vi "ShooterSpeedRegulateV2 Debug.vi"(0 "Shooter Speed":T2(ring)) -> (4 "ALL GOOD":bool, 10 "Motor 1 Output":dbl)   [LabVIEW 2012]
uses:
  Robot Global Data.vi
  Max'sToolKit/ConvertVoltageToPercentVbs.vi
  <vilib>/addons/control/pid/pid.llb/PID (DBL).vi
  <vilib>/addons/control/pid/NI_PID_pid.lvlib
panel:
  in  "Use PID":bool
  out "Waveform Chart":cluster{dbl, "upper limit":dbl, dbl}(graph)
  in  "Feed Foward \nVoltage":dbl format="%_6g"
  in  "PID gains":T1
  out "Motor Voltage":dbl
  out "Error":dbl
  in  "Reset Shooter PID":bool
  out "Loop Rate (Hz)":dbl
  out "Array Index":dbl
  out "Wheel 1 RPS":dbl
  out "W1 Target RPS":dbl
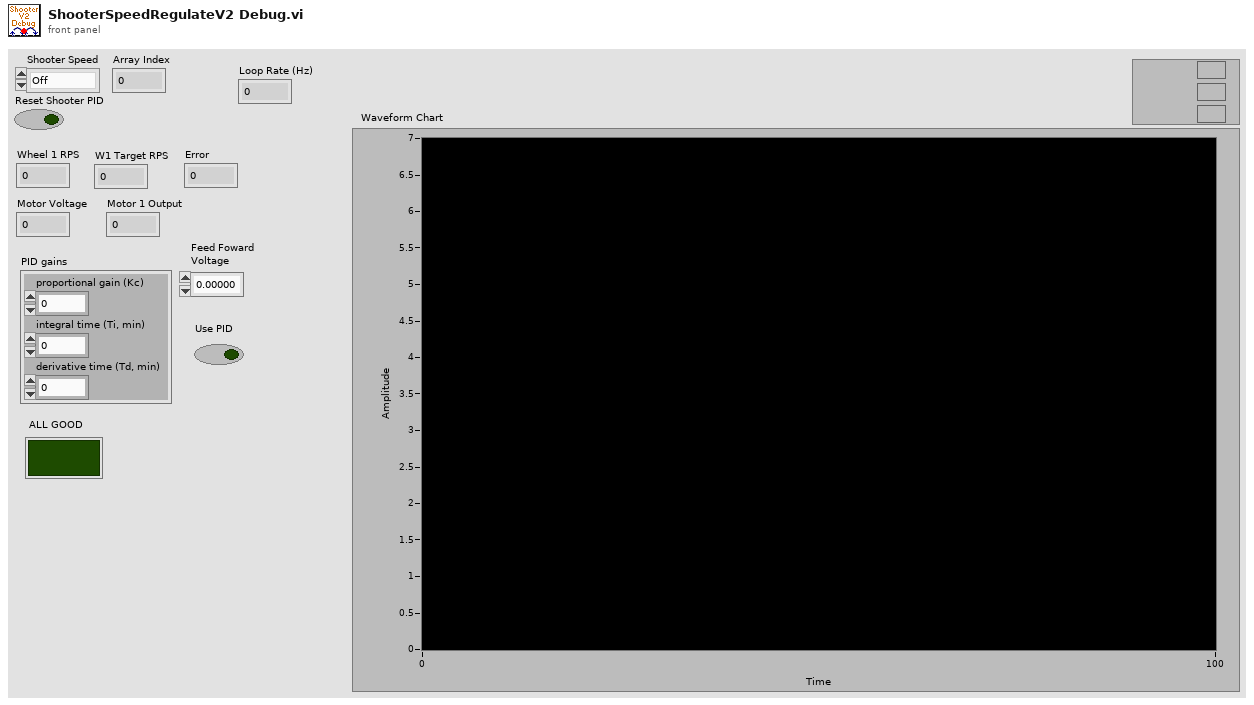
[diagram p1: front panel]
types:
  T1 = cluster{"proportional gain (Kc)":dbl, "integral time (Ti, min)":dbl, "derivative time (Td, min)":dbl}
  T2 = enum16{"Off", "2pt Key Shot", "3pt Key Shot", "Back Shot", "Fender Shot", "Key Close", "Key Far"}
  T3 = typedef "WPI_EncoderDevRef.ctl" = cluster{"DevStatus":errorcluster, "EncoderIndex":T4, "CounterIndex":T5, "DistancePerCount":dbl, "Decoding Type":T6}
  T4 = typedef "FPGA_EncoderIdx.ctl" = enum8{"Enc 0", "Enc 1", "Enc 2", "Enc 3", "Invalid"}
  T5 = typedef "FPGA_CounterCtrSystemIndex.ctl" = enum8{"Ctr 0", "Ctr 1", "Ctr 2", "Ctr 3", "Ctr 4", "Ctr 5", "Ctr 6", "Ctr 7", "Invalid"}
  T6 = typedef "WPI_EncoderType.ctl" = enum16{"1x", "2x", "4x"}
  T7 = typedef "WPI_MotorControlDeviceRef.ctl" = cluster{"DeviceStatus":errorcluster, "Type":enum16{"PWM", "CAN"}, "PWM":cluster{"Digital Module":T8, "PWM Channel":T9, "DeadBand":T10}, "CAN":cluster{"Device Number":u8, "Control Mode":T11, "Semaphore":T12, "Max Vout":dbl}, "Invert":bool, "TransformRef":T13, "InvTransformRef":T13}
  T8 = typedef "FPGA_TypedefDigitalModule.ctl" = enum16{"Digital Module 1", "Digital Module 2"}
  T9 = typedef "FPGA_DIOPWMChannel.ctl" = enum8{"PWM 1", "PWM 2", "PWM 3", "PWM 4", "PWM 5", "PWM 6", "PWM 7", "PWM 8", "PWM 9", "PWM 10", "Invalid"}
  T10 = typedef "WPI_PWMDeadband.ctl" = cluster{"Name":string, "maxPositivePwm":i32, "minPositivePwm":i32, "centerPwm":i32, "maxNegativePwm":i32, "minNegativePwm":i32, "angularRange":u16}
  T11 = typedef "WPI_CANJaguar_ControlMode.ctl" = enum8{"Percent VBus", "Current", "Speed", "Position", "Voltage"}
  T12 = typedef "Semaphore RefNum" = refnum<k1>
  T13 = typedef "WPI_PWMTransform_ConPane.ctl" = refnum<vi>
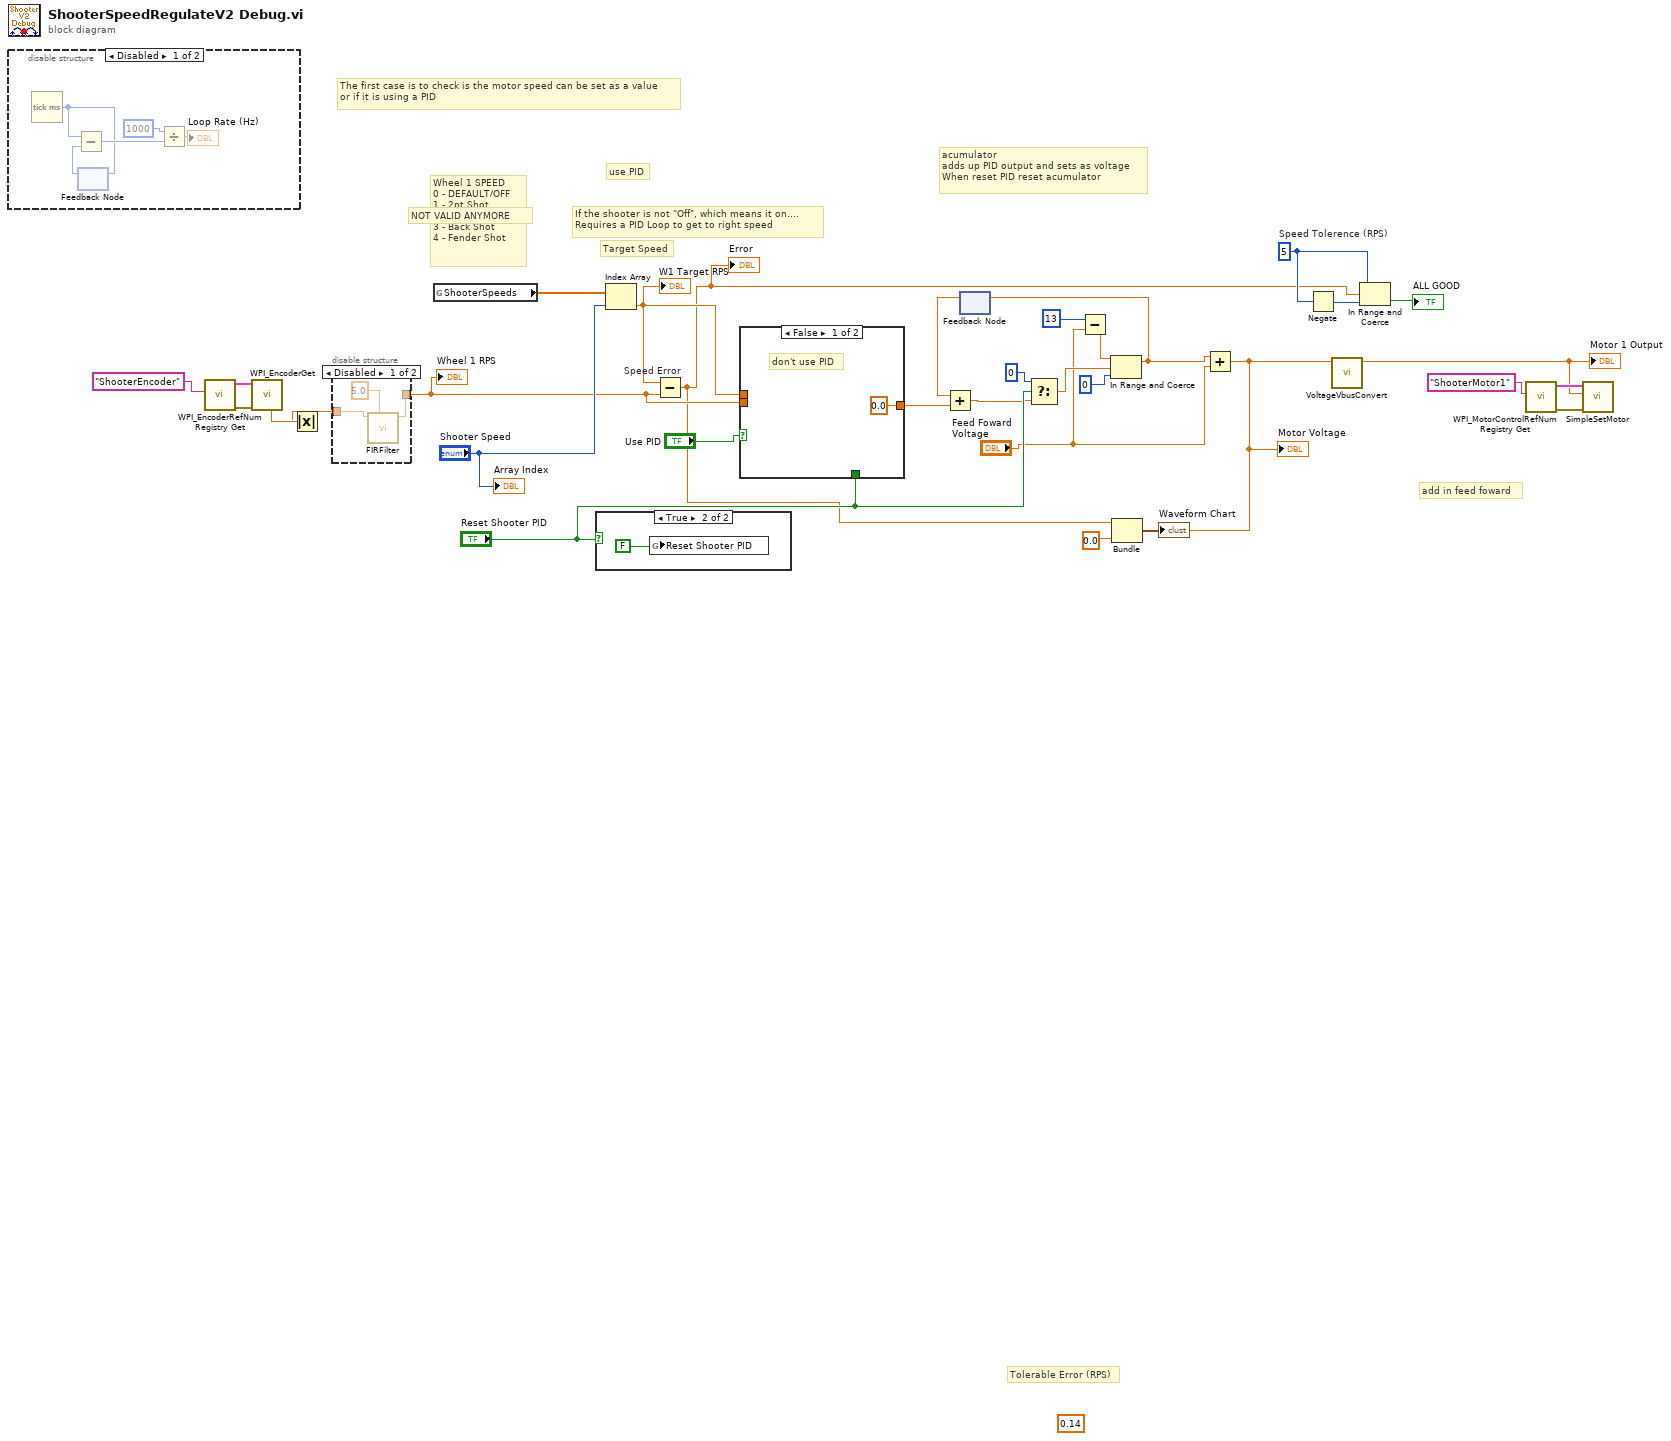
[diagram p0: block diagram]
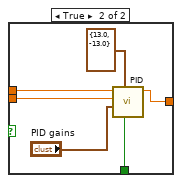
[diagram p2: hidden frame]
diagram:
  w18 = 5  # Speed Tolerence (RPS)
  (unwired) 0.14
  # "add in feed foward"
  # "acumulator\nadds up PID output and sets as voltage\nWhen reset PID reset acumulator"
  # "Target Speed"
  # "If the shooter is not \"Off\", which means it on....\nRequires a PID Loop to get to right speed"
  # "use PID"
  # "NOT VALID ANYMORE"
  # "The first case is to check is the motor speed can be set as a value\nor if it is using a PID"
  # "Tolerable Error (RPS)"
  # "Wheel 1 SPEED\n0 - DEFAULT/OFF\n1 - 2pt Shot\n2 - 3pt Key Shot\n3 - Back Shot\n4 - Fender Shot"
  n1 = disable-structure shown="Disabled" {
    frame Disabled {
      n2 = Tick Count (ms)() -> (millisecond timer value=w33:u32)
      n3 = feedback #1() -> (w34:u32)  [unwired: 1 in]
      n4 = Subtract(x=w33, y=w34) -> (x-y=w36:u32)
      n5 = feedback-in #1(w33) -> ()
      n6 = Divide(x=1000, y=w36) -> (x/y=→"Loop Rate (Hz)":dbl)
    }
    frame Enabled {
    }
  }
  n7 = call <vilib>:"WPI_EncoderRefNum Registry Get.vi"("refnum name"="ShooterEncoder") -> ("error out"=w25:errorcluster, "EncoderDevRef"=w26:T3)  [unwired: 9 in]
  n8 = call <vilib>:"WPI_EncoderGet.vi"("error in (no error)"=w25, "EncoderDevRef"=w26) -> ("Rate"=w22:dbl)  [unwired: 4 in, 5 out]
  n9 = Absolute Value(x=w22) -> (abs(x)=w21:dbl)
  n10 = disable-structure shown="Disabled" {
    disable-tunnel: [w39 w41] -> w24
    disable-tunnel: w21 -> [w38 w41]
    frame Disabled {
      n11 = call "FIRFilter.vi"("Filter Size"=5.0 ("Filter size"), "Input"=w38) -> ("Output"=w39:dbl)  [unwired: 9 in]
    }
    frame Enabled {
    }
  }
  "Wheel 1 RPS" <- w24
  n12 = global read "Robot Global Data.vi" "ShooterSpeeds"() -> (w23:dbl[])
  n13 = case shown="True" "Reset Shooter PID" {
    frame False {
    }
    frame True {
      n14 = global write "Robot Global Data.vi" "Reset Shooter PID"(FALSE) -> ()
    }
  }
  n15 = Index Array(array=w23, index="Shooter Speed") -> (element=w13:dbl)
  "W1 Target RPS" <- w13
  n16 = Subtract "Speed Error"(x=w13, y=w24) -> (x-y=w10:dbl)
  "Error" <- w10
  n17 = case shown="False" "Use PID" {
    tunnel: w24 -> [_ w49]
    tunnel: "Reset Shooter PID" -> [_ w48]
    tunnel: w13 -> [_ w45]
    tunnel: [0.0 ("output") w44] -> w12
    frame False {
      # "don't use PID"
    }
    frame True {
      n18 = call-poly <vilib>:"PID.vi"("reinitialize? (F)"=w48, "output range"=cluster{"output high":dbl, "output low":dbl} {"output high"=13.0, "output low"=-13.0}, "PID gains"="PID gains", "process variable"=w49, "setpoint"=w45) -> ("output"=w44:dbl)  [unwired: 5 in, 1 out]
    }
  }
  n19 = feedback #2() -> (w14:dbl)  [unwired: 1 in]
  n20 = Add(x=w14, y=w12) -> (x+y=w6:dbl)
  n21 = Select(t=0, s="Reset Shooter PID", f=w6) -> (s? t:f=w11:dbl)
  n22 = Subtract(x=13 ("upper limit"), y="Feed Foward \nVoltage") -> (x-y=w4:dbl)
  n23 = In Range and Coerce(upper limit=w4, x=w11, lower limit=0 ("upper limit")) -> (coerced(x)=w3:dbl)  [unwired: 1 out]
  n24 = feedback-in #2(w3) -> ()
  n25 = Add(x=w3, y="Feed Foward \nVoltage") -> (x+y=w2:dbl)
  "Motor Voltage" <- w2
  n26 = Bundle(w10, w2, 0.0) -> (→"Waveform Chart":cluster{dbl, dbl, dbl})  [unwired: 1 in]
  n27 = Negate(x=w18) -> (-x=w28:i32)
  n28 = call-poly "VoltageVbusConvert.vi"("Voltage"=w2) -> ("Vbus"=w17:dbl)  [unwired: 10 in]
  "Motor 1 Output" <- w17
  n29 = In Range and Coerce(upper limit=w18, x=w10, lower limit=w28) -> (In Range?=→"ALL GOOD":bool)  [unwired: 1 out]
  n30 = call <vilib>:"WPI_MotorControlRefNum Registry Get.vi"("refnum name"="ShooterMotor1") -> ("error out"=w30:errorcluster, "MotorControlDevRef"=w31:T7)  [unwired: 9 in]
  n31 = call "SimpleSetMotor.vi"("error in (no error)"=w30, "Output"=w17, "MotorControlDevRef"=w31) -> ()  [unwired: 7 in, 2 out]
  "Array Index" <- "Shooter Speed"
